vi "writeToXML.vi"(8 "error in (no error)":errorcluster, 10 "ClassLabel":string, 11 "CollOffset in":refnum<class "CollOffset.lvclass">) -> (0 "error out":errorcluster, 2 "XML out":string, 3 "CollOffset out":refnum<class "CollOffset.lvclass">)   [LabVIEW 2022 SP3, in "TCSDataDefinitions.lvlib" / "TCSCommand.lvlib" / "OffsetCommands.lvlib" / "CollOffset.lvclass"]
uses:
  CollOffset.lvclass
  <userlib>/Common/UnitsAndXML/FlattenItemWithUnitToXML/FlattenPlaneAngleToXML/PlaneAngleUnit.ctl
  CollOffset.lvclass/CollOffset.ctl
  CollimationOffsetCommands/CollimationOffsetCommands.lvclass
  <userlib>/Common/UnitsAndXML/UnitsAndXML.lvlib
  <userlib>/Common/XML/XMLGenerator/XMLGenerator.lvclass
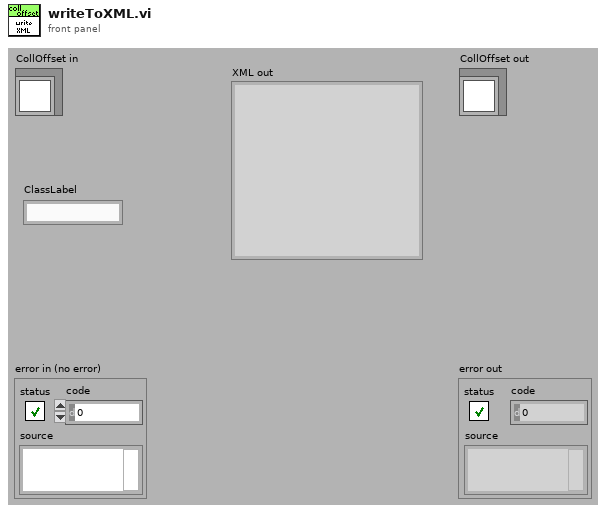
[diagram p1: front panel]
types:
  T1 = typedef "UnitsAndXML.lvlib/PlaneAngleUnit.ctl" = enum16{"rad", "deg", "'", "\""}
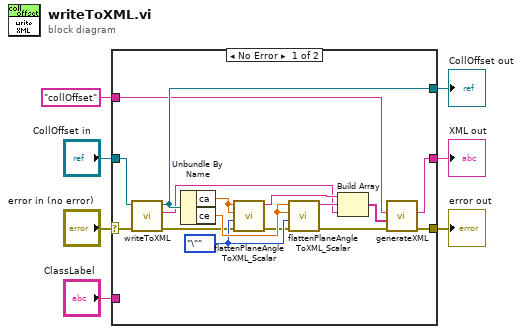
[diagram p0: block diagram]
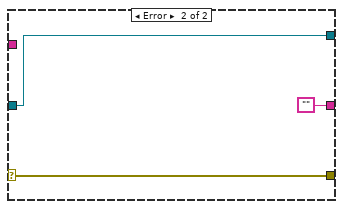
[diagram p2: hidden frame]
diagram:
  n1 = case shown="No Error" "error in (no error)" {
    selector: "error in (no error)" -> [w23 w26]
    tunnel: [w11 w26] -> w6
    tunnel: [w21 w25] -> w4
    tunnel: "CollOffset in" -> [w22 w25]
    tunnel: [w10 ""] -> w3
    tunnel: "collOffset" ("ClassLabel") -> [w8 _]
    tunnel: "ClassLabel" -> [_ _]
    frame No Error {
      w18 = PlaneAngleUnit."\"" ("planeAngleUnitInXML")
      n2 = call-parent "writeToXML.vi"("error in (no error)"=w23, "CollimationOffsetCommands in"=w22) -> ("error out"=w12:errorcluster, "XML out"=w9:string, "CollimationOffsetCommands out"=w21:refnum<class "CollOffset.lvclass">)  [unwired: 7 in]
      n3 = Unbundle By Name(w21) -> ("ca"=w20:dbl[unit], "ce"=w19:dbl[unit])
      n4 = call <userlib>:"flattenPlaneAngleToXML_Scalar.vi"("error in (no error)"=w12, "planeAngleUnitInXML"=w18, "planeAngleAgain"=w20, "planeAngle"=w20) -> ("error out"=w17:errorcluster, "xmlString"=w13:string)  [unwired: 6 in]
      n5 = call <userlib>:"flattenPlaneAngleToXML_Scalar.vi"("error in (no error)"=w17, "planeAngleUnitInXML"=w18, "planeAngleAgain"=w19, "planeAngle"=w19) -> ("error out"=w14:errorcluster, "xmlString"=w15:string)  [unwired: 6 in]
      n6 = Build Array(w13, w15, w9) -> (w16:string[])
      n7 = call <userlib>:"generateXML.vi"("error in"=w14, "childrenXML"=w16, "elementName"=w8) -> ("error out"=w11:errorcluster, "XML out"=w10:string)  [unwired: 6 in, 1 out]
    }
    frame Error {
    }
  }
  "error out" <- w6
  "CollOffset out" <- w4
  "XML out" <- w3
